vi "launch.vi"() -> ()   [LabVIEW 2016, in "工况数据上传.lvlib"]
uses:
  C:/Program Files (x86)/National Instruments/LabVIEW 2016/vi.lib/ActorFramework/Actor/Actor.lvclass
  <vilib>/ActorFramework/Message Enqueuer/Message Enqueuer.lvclass/Message Enqueuer.ctl
  <vilib>/ActorFramework/Message Enqueuer/Enqueue.vi
  <vilib>/ActorFramework/Stop Msg/Stop Msg.lvclass
  C:/Program Files (x86)/National Instruments/LabVIEW 2016/vi.lib/ActorFramework/Message/Message.lvclass
  <vilib>/ActorFramework/Message Priority Queue/Priority Enqueue.vi
  <vilib>/ActorFramework/Actor/Actor.lvclass
panel:
  in  "停止按钮":bool
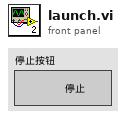
[diagram p1: front panel]
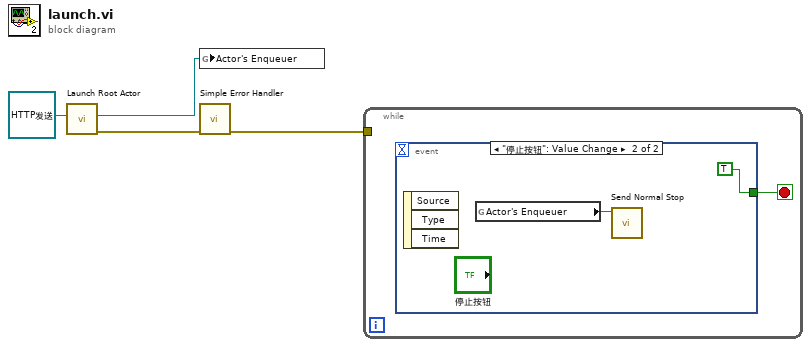
[diagram p0: block diagram]
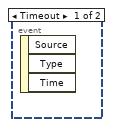
[diagram p2: hidden frame]
diagram:
  n1 = call <vilib>:"Launch Root Actor.vi"("Actor"=refnum<class "HTTP发送.lvclass"> refnum ("工况数据UI.lvlib:HTTP发送.lvclass")) -> ("error out"=w3:errorcluster, "Actor's Enqueuer"=w2:refnum<class "Message Enqueuer.lvclass">)  [unwired: 9 in]
  n2 = global write "工况数据接口全局.vi" "Actor's Enqueuer"(w2) -> ()
  n3 = call <vilib>:"Simple Error Handler.vi"("error in (no error)"=w3) -> ("error out"=w1:errorcluster)  [unwired: 4 in, 4 out]
  n4 = while {
    tunnel: w1 -> [_]
    stop <- w5 stop-if-true
    n5 = event shown="[1] \"停止按钮\": Value Change" {
      selector: _ -> [_ _]
      dyn-events: _ -> [_ _]
      timeout: _ -> [_ _]
      tunnel: [_ TRUE] -> w5
      event Timeout {
        n6 = event-data() -> ()  [unwired: 1 in, 3 out]
      }
      event "停止按钮": Value Change {
        n7 = event-data() -> ()  [unwired: 1 in, 3 out]
        n8 = global read "工况数据接口全局.vi" "Actor's Enqueuer"() -> (w7:refnum<class "Message Enqueuer.lvclass">)
        n9 = call <vilib>:"Send Normal Stop.vi"("Message Enqueuer"=w7) -> ()  [unwired: 10 in, 1 out]
      }
    }
  }
